vi "KeDSO Initiate Digitizing Process.vi"(8 "error in":errorcluster, 11 "keysight dso":T1 {"bw limit [Hz]" format="%#_6p"; "channels"."Offset [V]" min=0.0 format="%#_6p"; "channels"."Range [Vpk]" min=0.0 format="%#_6p"; "channels"."Channel" min=1}) -> (0 "error out":errorcluster, 3 "keysight dso out":T1 {"bw limit [Hz]" format="%#_6p"; "channels"."Offset [V]" min=0.0 format="%#_6p"; "channels"."Range [Vpk]" min=0.0 format="%#_6p"; "channels"."Channel" min=1})   [LabVIEW 2013]
doc: "Initiates digitizing process. Acquisition starts according trigger setup. Can be called repetitively for another record using current setup."
uses:
  KeDSO session.ctl
  KeDSO Virtual Channel.ctl
  KeDSO Trigger Setup.ctl
  KeDSO Trigger Source.ctl
  Agilent 90000 Series.lvlib
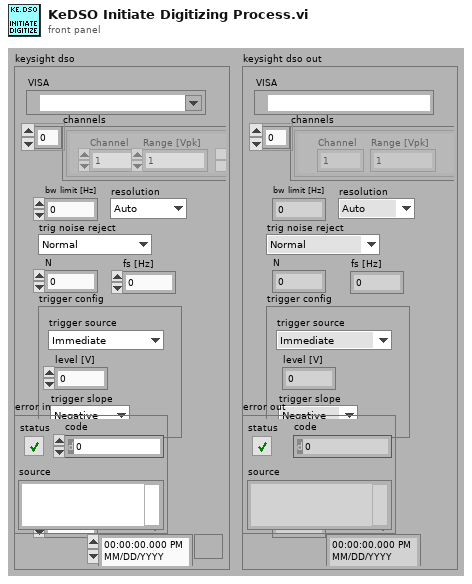
[diagram p1: front panel]
types:
  T1 = typedef "KeDSO session.ctl" = cluster{"VISA":refnum<visa-resource-name>, "channels":T2[], "bw limit [Hz]":dbl, "resolution":enum16{"Auto", "Bits 9", "Bits 10", "Bits 11", "Bits 12"}, "trig noise reject":enum16{"Normal", "High Sensitivity"}, "N":i64, "trigger config":T3, "fs [Hz]":dbl, "timeout stop":timestamp, "waiting for opc":bool, "fetch offset [smpl]":i64, "abs timestamp":timestamp}
  T2 = typedef "KeDSO Virtual Channel.ctl" = cluster{"Channel":i32, "Range [Vpk]":dbl, "btn clr":bool, "btn up":bool, "btn down":bool, "Offset [V]":dbl, "Coupling":enum16{"DC", "DC50", "AC", "LFR1"}, "bw limit enab":bool}
  T3 = typedef "KeDSO Trigger Setup.ctl" = cluster{"trigger source":T4, "level [V]":dbl, "trigger slope":enum16{"Negative", "Positive", "Either"}}
  T4 = typedef "KeDSO Trigger Source.ctl" = enum16{"Immediate", "Level", "AUX"}
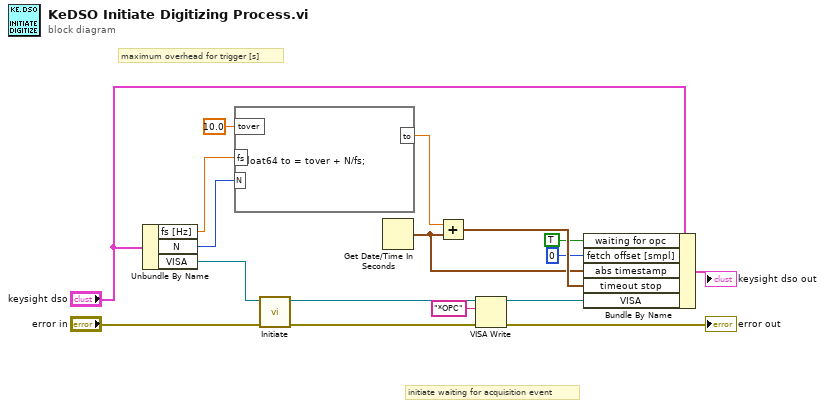
[diagram p0: block diagram]
diagram:
  # "initiate waiting for acquisition event"
  # "maximum overhead for trigger [s]"
  n1 = Unbundle By Name("keysight dso") -> ("fs [Hz]"=w12:dbl, "N"=w11:i64, "VISA"=w14:refnum<visa-resource-name>)
  n2 = formula code="float64 to = tover + N/fs;"("fs"=w12, "N"=w11, "tover"=10.0 ("input variable")) -> ("to"=w10:dbl)
  n3 = call "Initiate.vi"("error in (no error)"="error in", "VISA resource name"=w14) -> ("error out"=w7:errorcluster, "VISA resource name out"=w8:refnum<visa-resource-name>)  [unwired: 8 in]
  n4 = Get Date/Time In Seconds() -> (seconds since 1Jan1904=w3:timestamp)
  n5 = Add(x=w10, y=w3) -> (x+y=w9:timestamp)
  n6 = VISA Write(VISA resource name=w8, write buffer="*OPC", error in (no error)=w7) -> (VISA resource name out=w5:refnum<visa-resource-name>, error out=→"error out":errorcluster)  [unwired: 1 out]
  n7 = Bundle By Name(cluster="keysight dso", "waiting for opc"=TRUE, "fetch offset [smpl]"=i64 0, "abs timestamp"=w3, "timeout stop"=w9, "VISA"=w5) -> (→"keysight dso out":T1)
